vi "VERSION.vi"(8 "Software Version":u16=1, 9 "Hardware Version":u16=1, 11 "Python in":string) -> (3 "Python out":string="uart.write(b'\\x5F\\x01\\x00\\x00\\x00\\x01\\x00\\x00\\x00\\xA0')\n")   [LabVIEW 2016]
panel:
  out "bytes added":u8[](array[numeric])=[95, 1, 0, 0, 0, 1, 0, 0, 0, 160] format="%.0x"
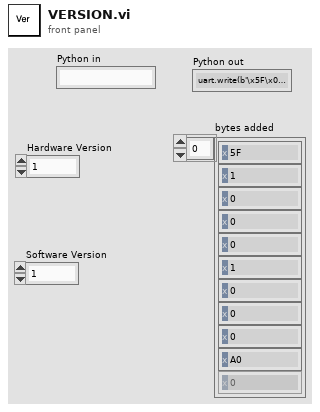
[diagram p1: front panel]
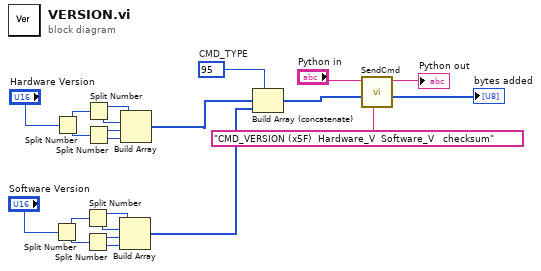
[diagram p0: block diagram]
diagram:
  w22 = u8 95  # CMD_TYPE
  n1 = Split Number(x="Software Version") -> (hi(x)=w6:u8, lo(x)=w5:u8)
  n2 = Split Number(x="Hardware Version") -> (hi(x)=w15:u8, lo(x)=w16:u8)
  n3 = Split Number(x=w6) -> (hi(x)=w7:u8, lo(x)=w8:u8)
  n4 = Split Number(x=w5) -> (hi(x)=w9:u8, lo(x)=w10:u8)
  n5 = Split Number(x=w15) -> (hi(x)=w14:u8, lo(x)=w13:u8)
  n6 = Split Number(x=w16) -> (hi(x)=w12:u8, lo(x)=w11:u8)
  n7 = Build Array(w7, w8, w9, w10) -> (w2:u8[])
  n8 = Build Array(w14, w13, w12, w11) -> (w3:u8[])
  n9 = Build Array (concatenate)(w22, w3, w2) -> (w19:u8[])
  n10 = call "SendCmd.vi"("Comment"="CMD_VERSION (x5F)  Hardware_V  Software_V   checksum", "Array In"=w19, "Python in"="Python in") -> ("Array Sent"=→"bytes added":u8[], "Python out"=→"Python out":string)  [unwired: 7 in]
